vi "Sample Timing.vi"(5 "dt":dbl, 7 "# Samples":i32, 10 "error in (no error)":errorcluster) -> (2 "error out":errorcluster, 3 "t0":timestamp)   [LabVIEW 2020, in "VolatusDAQ.lvlib"]
uses:
  VolatusDAQ.lvlib
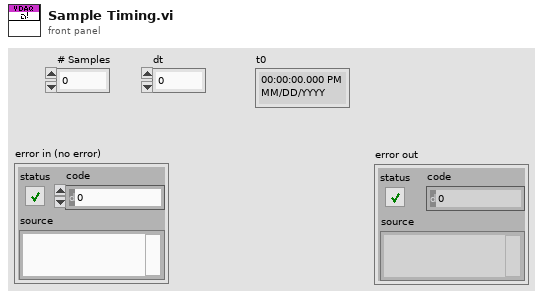
[diagram p1: front panel]
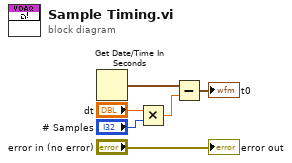
[diagram p0: block diagram]
diagram:
  n1 = Get Date/Time In Seconds() -> (seconds since 1Jan1904=w2:timestamp)
  n2 = Multiply(x="dt", y="# Samples") -> (x*y=w3:dbl)
  n3 = Subtract(x=w2, y=w3) -> (x-y=→"t0":timestamp)
  "error out" <- "error in (no error)"
